vi "Saving Img Data.vi"(8 "error in (no error)":errorcluster caption="错误输入（无错误）", 10 "Image":T1, 11 "名称或相对路径":string) -> (0 "error out":errorcluster caption="错误输出")   [LabVIEW 2015, in "Utility VIs.lvlib"]
uses:
  Utility VIs.lvlib
  <vilib>/vision/Image Controls.llb/IMAQ Image.ctl
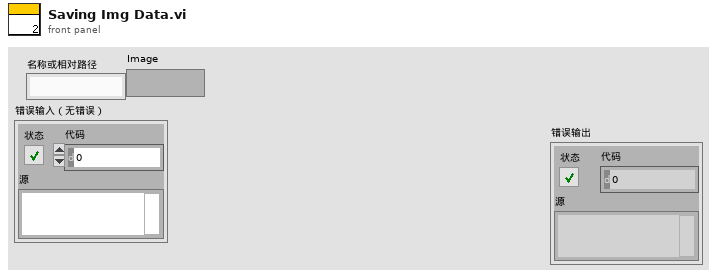
[diagram p1: front panel]
types:
  T1 = typedef "IMAQ Image.ctl" = refnum<image>
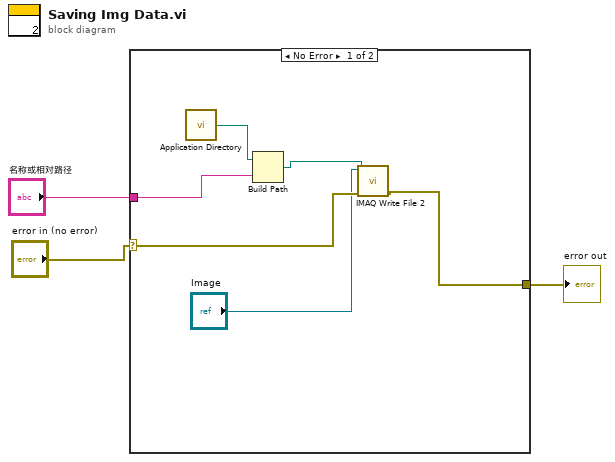
[diagram p0: block diagram]
diagram:
  n1 = case shown="No Error" "error in (no error)" {
    selector: "error in (no error)" -> [w6 w10]
    tunnel: "名称或相对路径" -> [w8 _]
    tunnel: [w7 w10] -> w2
    frame No Error {
      n2 = call <vilib>:"Application Directory.vi"() -> ("Application Directory"=w9:path)
      n3 = Build Path(base path=w9, name or relative path=w8) -> (appended path=w5:path)
      n4 = call-poly "IMAQ Write File 2"("error in (no error)"=w6, "File Path"=w5, "Image"="Image") -> ("error out"=w7:errorcluster)  [unwired: 7 in, 1 out]
    }
    frame Error {
    }
  }
  "error out" <- w2
